vi "GetADCTester (SubVI).vi"(8 "error in (no error)":errorcluster, 9 "GetADCTester":T1(ring), 10 "TimeToGet":i32, 11 "VISA Refnum in":refnum<visa-resource-name>) -> (0 "error out":errorcluster, 2 "ADCValOutput Single":u32, 3 "ADCValOutput Arr":u32[](array[numeric]))   [LabVIEW 2017]
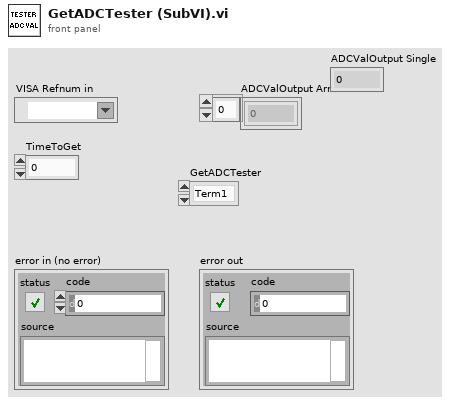
[diagram p1: front panel]
types:
  T1 = enum8{"Term1", "Term2", "Current", "Fan", "TempCPU"}
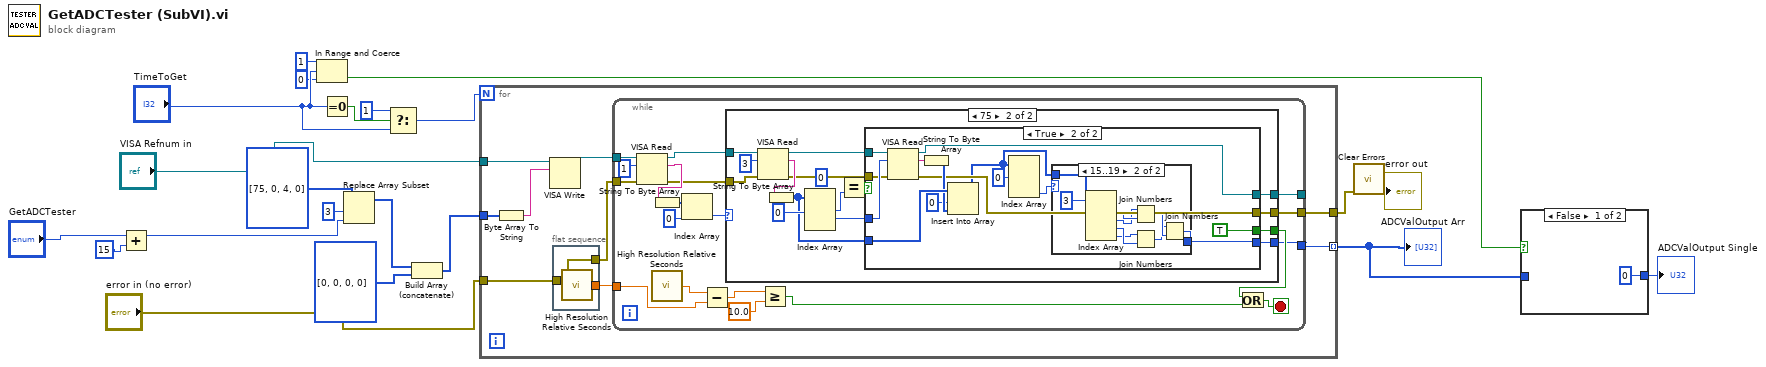
[diagram p0: block diagram]
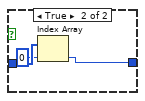
[diagram p2: hidden frame]
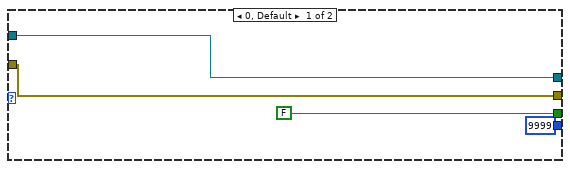
[diagram p3: hidden frame]
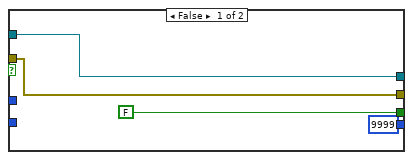
[diagram p4: hidden frame]
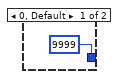
[diagram p5: hidden frame]
diagram:
  n1 = Add(x="GetADCTester", y=u8 15) -> (x+y=w3:u8)
  n2 = In Range and Coerce(upper limit=1, x="TimeToGet", lower limit=0) -> (In Range?=w6:bool)  [unwired: 1 out]
  n3 = Equal To 0?(x="TimeToGet") -> (x = 0?=w19:bool)
  n4 = Replace Array Subset(array=u8[] [75, 0, 4, 0], new element=w3, index=3) -> (w15:u8[])
  n5 = Select(t=1, s=w19, f="TimeToGet") -> (s? t:f=w20:i32)
  n6 = Build Array (concatenate)(w15, u8[] [0, 0, 0, 0]) -> (w16:u8[])
  n7 = for {
    N: w20 -> [_]
    tunnel: "VISA Refnum in" -> [w27]
    tunnel: w16 -> [w26]
    tunnel: [w24] -> w7 mode=indexing
    tunnel: "error in (no error)" -> [w23]
    tunnel: [w25] -> w17
    n8 = Byte Array To String(unsigned byte array=w26) -> (string=w30:string)
    n9 = VISA Write(VISA resource name=w27, write buffer=w30) -> (VISA resource name out=w28:refnum<visa-resource-name>)  [unwired: 1 in, 2 out]
    n10 = flat-sequence {
      tunnel: [w32] -> w29
      tunnel: w23 -> [w31]
      tunnel: [w31] -> w22
      frame #0 {
        n11 = call <vilib>:"High Resolution Relative Seconds.vi"() -> ("relative seconds"=w32:dbl)
      }
    }
    n12 = while {
      tunnel: w28 -> [w44]
      tunnel: w22 -> [w43]
      tunnel: [w42] -> _
      tunnel: [w41] -> w25
      tunnel: w29 -> [w37]
      tunnel: [w33] -> w24
      stop <- w40 stop-if-true
      n13 = VISA Read(VISA resource name=w44, byte count=u32 1, error in (no error)=w43) -> (VISA resource name out=w46:refnum<visa-resource-name>, read buffer=w47:string, error out=w45:errorcluster)  [unwired: 1 out]
      n14 = String To Byte Array(string=w47) -> (unsigned byte array=w50:u8[])
      n15 = call <vilib>:"High Resolution Relative Seconds.vi"() -> ("relative seconds"=w38:dbl)
      n16 = Index Array(array=w50, index=0) -> (element=w48:u8)
      n17 = Subtract(x=w38, y=w37) -> (x-y=w36:dbl)
      n18 = case shown="75" w48 {
        tunnel: [w55 w59] -> w41
        tunnel: w46 -> [w54 w68]
        tunnel: w45 -> [w55 w67]
        tunnel: [w54 w60] -> w42
        tunnel: [FALSE w57] -> w39
        tunnel: [u32 9999 w56] -> w33
        frame 0, Default {
        }
        frame 75 {
          n19 = VISA Read(VISA resource name=w68, byte count=u32 3, error in (no error)=w67) -> (VISA resource name out=w63:refnum<visa-resource-name>, read buffer=w71:string, error out=w62:errorcluster)  [unwired: 1 out]
          n20 = String To Byte Array(string=w71) -> (unsigned byte array=w61:u8[])
          n21 = Index Array(array=w61, index #1=0 ("index")) -> (element #1=w66:u8, element #2=w64:u8)  [unwired: 2 in, 1 out]
          n22 = Equal?(x=u8 0, y=w66) -> (x = y?=w65:bool)
          n23 = case shown="True" w65 {
            tunnel: [w74 w82] -> w59
            tunnel: w64 -> [_ w89]
            tunnel: w63 -> [w75 w88]
            tunnel: w62 -> [w74 w87]
            tunnel: w61 -> [_ w86]
            tunnel: [w75 w84] -> w60
            tunnel: [FALSE TRUE] -> w57
            tunnel: [u32 9999 w76] -> w56
            frame False {
            }
            frame True {
              n24 = VISA Read(VISA resource name=w88, byte count=w89, error in (no error)=w87) -> (VISA resource name out=w84:refnum<visa-resource-name>, read buffer=w83:string, error out=w82:errorcluster)  [unwired: 1 out]
              n25 = String To Byte Array(string=w83) -> (unsigned byte array=w85:u8[])
              n26 = Insert Into Array(array=w86, index=0, new element=w85) -> (w77:u8[])
              n27 = Index Array(array=w77, index #1=0 ("index")) -> (element #3=w78:u8)  [unwired: 2 in, 2 out]
              n28 = case shown="15..19" w78 {
                tunnel: w77 -> [_ w98]
                tunnel: [u32 9999 w91] -> w76
                frame 0, Default {
                }
                frame 15..19 {
                  n29 = Index Array(array=w98, index #1=3 ("index")) -> (element #1=w97:u8, element #2=w96:u8, element #3=w95:u8, element #4=w94:u8)  [unwired: 3 in]
                  n30 = Join Numbers(hi=w96, lo=w97) -> ((hi.lo)=w93:u16)
                  n31 = Join Numbers(hi=w94, lo=w95) -> ((hi.lo)=w92:u16)
                  n32 = Join Numbers(hi=w92, lo=w93) -> ((hi.lo)=w91:u32)
                }
              }
            }
          }
        }
      }
      n33 = Greater Or Equal?(x=w36, y=10.0) -> (x >= y?=w34:bool)
      n34 = Or(x=w39, y=w34) -> (x .or. y?=w40:bool)
    }
  }
  "ADCValOutput Arr" <- w7
  n35 = call <vilib>:"Clear Errors.vi"("error in (no error)"=w17) -> ("error out"=→"error out":errorcluster)  [unwired: 5 in, 1 out]
  n36 = case shown="False" w6 {
    tunnel: w7 -> [_ w103]
    tunnel: [u32 0 w101] -> w5
    frame False {
    }
    frame True {
      n37 = Index Array(array=w103, index=0) -> (element=w101:u32)
    }
  }
  "ADCValOutput Single" <- w5
